vi "PrepLineObjectArray_size.vi"(8 "error in (no error)":errorcluster) -> (0 "error out":errorcluster, 2 "size(s)":i32)   [LabVIEW 2017]
doc: "Return the size (number of elements) of the PrepLineObject Array"
uses:
  global variables.vi
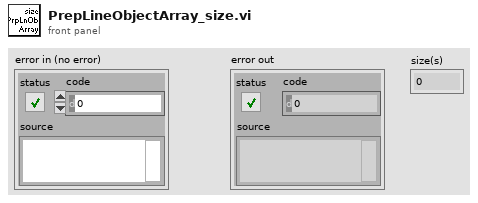
[diagram p1: front panel]
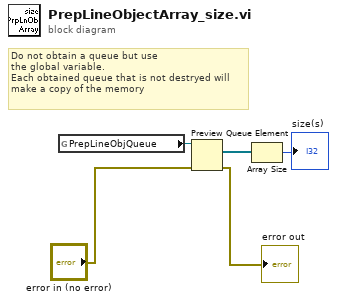
[diagram p0: block diagram]
diagram:
  # "Do not obtain a queue but use\nthe global variable.\nEach obtained queue that is not destryed will\nmake a copy of the memory"
  n1 = global read "global variables.vi" "PrepLineObjQueue"() -> (w5:refnum<queue>)
  n2 = Preview Queue Element(queue=w5, error in (no error)="error in (no error)") -> (element=w2:refnum<class "PrepLineObject.lvclass">[], error out=→"error out":errorcluster)  [unwired: 1 in, 2 out]
  n3 = Array Size(array=w2) -> (size(s)=→"size(s)":i32)
